vi "Integrate.vi"(1 "Array":dbl[](array[numeric])) -> (0 "Integral result":dbl)   [LabVIEW 2014]
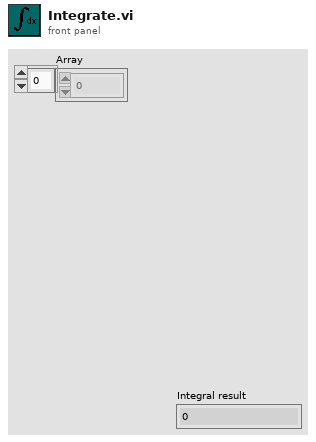
[diagram p1: front panel]
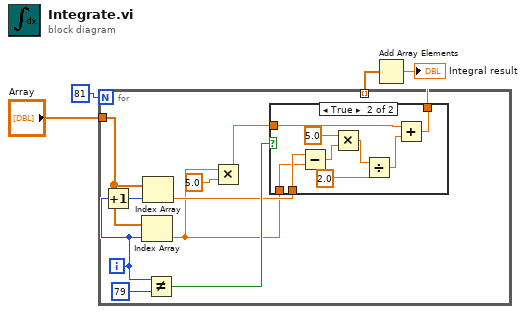
[diagram p0: block diagram]
diagram:
  n1 = for {
    N: 81 -> [_]
    tunnel: [w14] -> w2 mode=indexing
    tunnel: "Array" -> [w10]
    i -> [w9]
    n2 = Increment(x=w9) -> (x+1=w8:i32)
    n3 = Index Array(array=w10, index=w9) -> (element=w5:dbl)
    n4 = Index Array(array=w10, index=w8) -> (element=w6:dbl)
    n5 = Not Equal?(x=w9, y=79) -> (x != y?=w11:bool)
    n6 = Multiply(x=w5, y=5.0) -> (x*y=w7:dbl)
    n7 = case shown="True" w11 {
      tunnel: w7 -> [w15 w20]
      tunnel: [w15 w19] -> w14
      tunnel: w6 -> [_ w18]
      tunnel: w5 -> [_ w17]
      frame False {
      }
      frame True {
        n8 = Subtract(x=w18, y=w17) -> (x-y=w24:dbl)
        n9 = Multiply(x=5.0, y=w24) -> (x*y=w23:dbl)
        n10 = Divide(x=w23, y=2.0) -> (x/y=w21:dbl)
        n11 = Add(x=w20, y=w21) -> (x+y=w19:dbl)
      }
    }
  }
  n12 = Add Array Elements(numeric array=w2) -> (sum=→"Integral result":dbl)
